vi "TurnCalculator.vi"(3 "Measured Coordinates (mm)":dbl[](array[numeric]), 5 "Top Left Corner Desired Coordinates (mm)":dbl[](array[numeric])) -> ()   [LabVIEW 2016]
uses:
  <vilib>/Analysis/baseanly.llb/Mean (DBL).vi
  <vilib>/Analysis/NI_AALBase.lvlib
panel:
  out "Y Knob Rotations":dbl
  out "X Knob Rotations":dbl
  out "Y displacement (microns)":dbl
  out "X displacement (microns)":dbl
  out "Angle Knob Rotations":dbl
  out "Radians from Ideal":dbl format="%0.5f"
  in  "Degrees per Rotation Angle":dbl format="%#_13g"
  in  "Microns per Rotation Y":dbl format="%#_13g"
  in  "Microns per Rotation X":dbl format="%#_13g"
  in  "Y Side length (m)":dbl=0.1 format="%#_13g"
  in  "X Side length (m)":dbl=0.1 format="%#_13g"
  in  "Desired Angle":dbl=0.026 format="%#_13g"
  # "Inputs"
  # "Outputs"
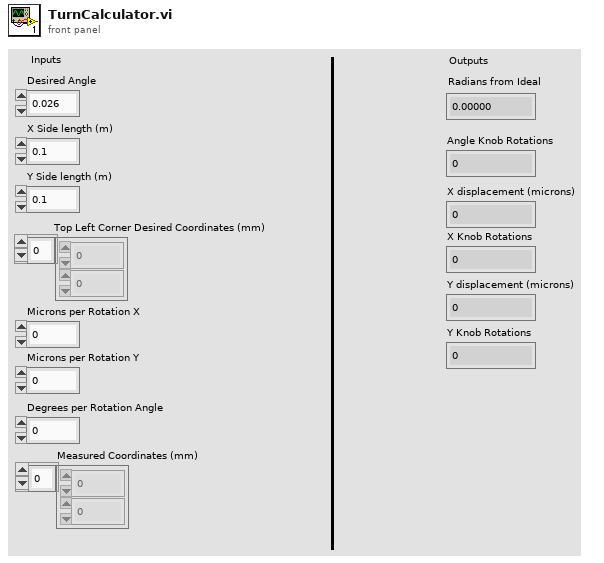
[diagram p1: front panel]
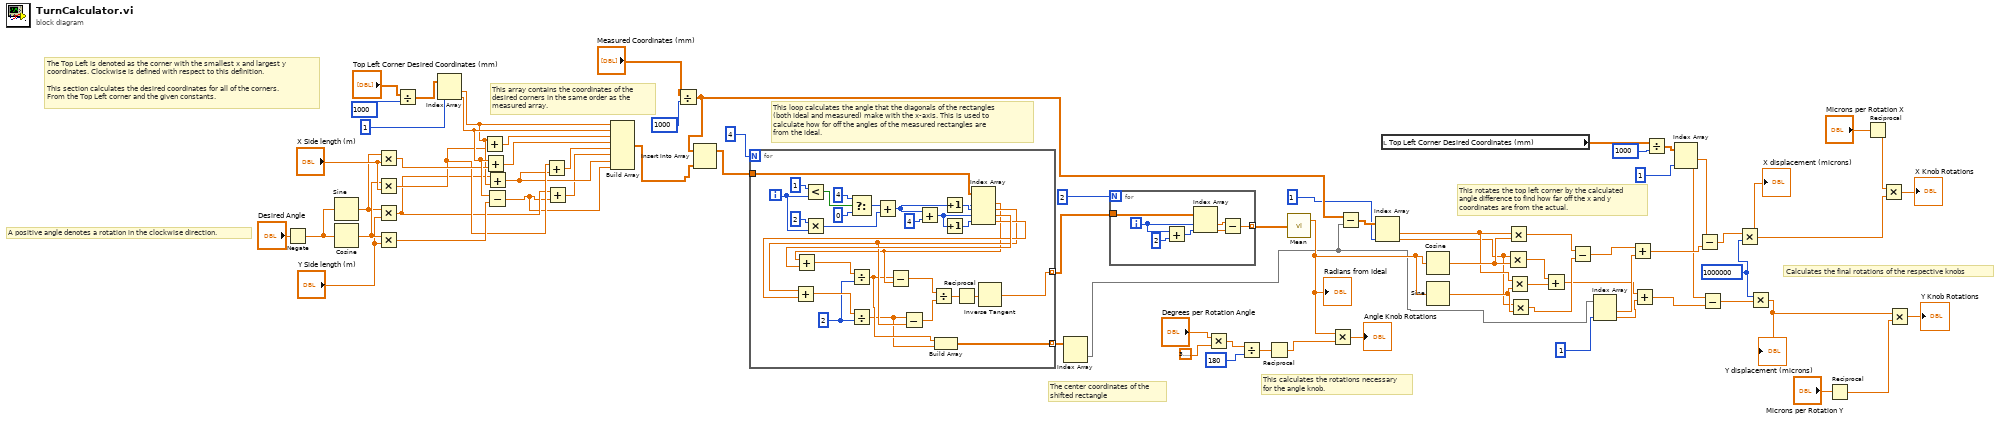
[diagram p0: block diagram]
diagram:
  w13 = 1000000
  # "Calculates the final rotations of the respective knobs"
  # "This rotates the top left corner by the calculated\nangle difference to find how far off the x and y \ncoordinates are from the actual."
  # "This calculates the rotations necessary\nfor the angle knob."
  # "The center coordinates of the\nshifted rectangle"
  # "This loop calculates the angle that the diagonals of the rectangles\n(both ideal and measured) make with the x-axis. This is used to\ncalculate how for off the angles of the measured rectangles are\nfrom the ideal."
  # "This array contains the coordinates of the\ndesired corners in the same order as the\nmeasured array."
  # "The Top Left is denoted as the corner with the smallest x and largest y\ncoordinates. Clockwise is defined with respect to this definition.\n\nThis section calculates the desired coordinates for all of the corners.\nFrom the Top Left corner and the given constants."
  # "A positive angle denotes a rotation in the clockwise direction."
  n1 = Negate(x="Desired Angle") -> (-x=w63:dbl)
  n2 = Sine(x=w63) -> (sin(x)=w71:dbl)
  n3 = Cosine(x=w63) -> (cos(x)=w72:dbl)
  n4 = Multiply(x=w71, y="X Side length (m)") -> (x*y=w65:dbl)
  n5 = Multiply(x=w72, y="X Side length (m)") -> (x*y=w62:dbl)
  n6 = Multiply(x=w71, y="Y Side length (m)") -> (x*y=w61:dbl)
  n7 = Multiply(x=w72, y="Y Side length (m)") -> (x*y=w67:dbl)
  n8 = Divide(x="Top Left Corner Desired Coordinates (mm)", y=1000) -> (x/y=w55:dbl[])
  n9 = Index Array(array=w55, index #2=1 ("index")) -> (element #1=w64:dbl, element #2=w66:dbl)  [unwired: 1 in]
  n10 = Add(x=w64, y=w62) -> (x+y=w69:dbl)
  n11 = Add(x=w66, y=w65) -> (x+y=w68:dbl)
  n12 = Subtract(x=w66, y=w67) -> (x-y=w50:dbl)
  n13 = Add(x=w61, y=w64) -> (x+y=w59:dbl)
  n14 = Add(x=w62, y=w59) -> (x+y=w49:dbl)
  n15 = Add(x=w61, y=w50) -> (x+y=w48:dbl)
  n16 = Build Array(w64, w66, w69, w68, w49, w48, w59, w50) -> (w58:dbl[])
  n17 = Divide(x="Measured Coordinates (mm)", y=1000) -> (x/y=w37:dbl[])
  n18 = Insert Into Array(array=w37, new element=w58) -> (w57:dbl[])  [unwired: 1 in]
  n19 = for {
    N: 4 -> [_]
    tunnel: w57 -> [w104]
    tunnel: [w79] -> w52 mode=indexing
    tunnel: [w76] -> w38 mode=indexing
    i -> [w95]
    w87 = 2
    n20 = Less?(x=1, y=w95) -> (x < y?=w93:bool)
    n21 = Multiply(x=2, y=w95) -> (x*y=w92:i32)
    n22 = Select(t=4, s=w93, f=0) -> (s? t:f=w97:i32)
    n23 = Add(x=w97, y=w92) -> (x+y=w80:i32)
    n24 = Add(x=w80, y=4) -> (x+y=w102:i32)
    n25 = Increment(x=w80) -> (x+1=w101:i32)
    n26 = Increment(x=w102) -> (x+1=w103:i32)
    n27 = Index Array(array=w104, index #1=w80, index #2=w101, index #3=w102, index #4=w103) -> (element #1=w81:dbl, element #2=w86:dbl, element #3=w91:dbl, element #4=w90:dbl)
    n28 = Add(x=w86, y=w90) -> (x+y=w89:dbl)
    n29 = Add(x=w81, y=w91) -> (x+y=w88:dbl)
    n30 = Divide(x=w88, y=w87) -> (x/y=w78:dbl)
    n31 = Divide(x=w89, y=w87) -> (x/y=w77:dbl)
    n32 = Subtract(x=w78, y=w81) -> (x-y=w84:dbl)
    n33 = Subtract(x=w77, y=w86) -> (x-y=w85:dbl)
    n34 = Divide(x=w84, y=w85) -> (x/y=w83:dbl)
    n35 = Build Array(w78, w77) -> (w76:dbl[])
    n36 = Reciprocal(x=w83) -> (1/x=w82:dbl)
    n37 = Inverse Tangent(1:w82) -> (0:w79:dbl)
  }
  n38 = Index Array(array=w38) -> (element=w24:dbl[])  [unwired: 2 in]
  n39 = for {
    N: 2 -> [_]
    tunnel: w52 -> [w111]
    tunnel: [w105] -> w47 mode=indexing
    i -> [w109]
    n40 = Add(x=w109, y=2) -> (x+y=w110:i32)
    n41 = Index Array(array=w111, index #1=w109, index #2=w110) -> (element #1=w107:dbl, element #2=w106:dbl)
    n42 = Subtract(x=w107, y=w106) -> (x-y=w105:dbl)
  }
  n43 = Multiply(x="Degrees per Rotation Angle", y=3.141592653589793) -> (x*y=w43:dbl)
  n44 = Divide(x=w43, y=180) -> (x/y=w41:dbl)
  n45 = Reciprocal(x=w41) -> (1/x=w40:dbl)
  n46 = call-poly <vilib>:"Mean.vi"("X"=w47) -> ("mean"=w34:dbl)  [unwired: 1 out]
  "Radians from Ideal" <- w34
  n47 = Multiply(x=w34, y=w40) -> (x*y=→"Angle Knob Rotations":dbl)
  n48 = Subtract(x=w37, y=w24) -> (x-y=w36:dbl[])
  n49 = Index Array(array=w36, index #2=1) -> (element #1=w31:dbl, element #2=w30:dbl)  [unwired: 1 in]
  n50 = local read "Top Left Corner Desired Coordinates (mm)"() -> (w3:dbl[])
  n51 = Cosine(x=w34) -> (cos(x)=w33:dbl)
  n52 = Sine(x=w34) -> (sin(x)=w32:dbl)
  n53 = Multiply(x=w30, y=w33) -> (x*y=w28:dbl)
  n54 = Multiply(x=w31, y=w33) -> (x*y=w26:dbl)
  n55 = Multiply(x=w31, y=w32) -> (x*y=w29:dbl)
  n56 = Multiply(x=w30, y=w32) -> (x*y=w27:dbl)
  n57 = Add(x=w28, y=w29) -> (x+y=w20:dbl)
  n58 = Subtract(x=w26, y=w27) -> (x-y=w21:dbl)
  n59 = Index Array(array=w24, index #2=1) -> (element #1=w22:dbl, element #2=w19:dbl)  [unwired: 1 in]
  n60 = Add(x=w21, y=w22) -> (x+y=w17:dbl)
  n61 = Add(x=w20, y=w19) -> (x+y=w15:dbl)
  n62 = Divide(x=w3, y=1000) -> (x/y=w1:dbl[])
  n63 = Index Array(array=w1, index #2=1) -> (element #1=w18:dbl, element #2=w16:dbl)  [unwired: 1 in]
  n64 = Subtract(x=w18, y=w17) -> (x-y=w14:dbl)
  n65 = Subtract(x=w16, y=w15) -> (x-y=w12:dbl)
  n66 = Multiply(x=w14, y=w13) -> (x*y=w6:dbl)
  "X displacement (microns)" <- w6
  n67 = Multiply(x=w13, y=w12) -> (x*y=w8:dbl)
  "Y displacement (microns)" <- w8
  n68 = Reciprocal(x="Microns per Rotation Y") -> (1/x=w9:dbl)
  n69 = Reciprocal(x="Microns per Rotation X") -> (1/x=w7:dbl)
  n70 = Multiply(x=w7, y=w6) -> (x*y=→"X Knob Rotations":dbl)
  n71 = Multiply(x=w8, y=w9) -> (x*y=→"Y Knob Rotations":dbl)
